vi "Moving Average Stacked Registers While Loop.vi"() -> ()   [LabVIEW 2023]
panel:
  out "Moving Average":dbl
  out "Current Value":dbl
  in  "stop":bool
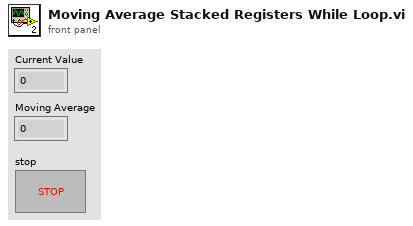
[diagram p1: front panel]
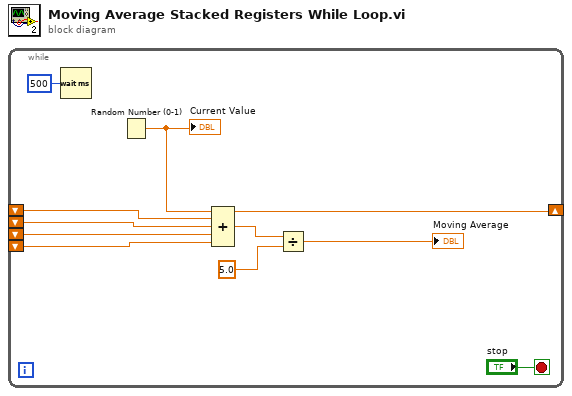
[diagram p0: block diagram]
diagram:
  n1 = while {
    shift-right: [w4] -> _
    shift-left: _ -> [w8]
    shift-left: _ -> [w6]
    shift-left: _ -> [w7]
    shift-left: _ -> [w5]
    stop <- "stop" stop-if-true
    n2 = Wait (ms)(milliseconds to wait=u32 500) -> ()  [unwired: 1 out]
    n3 = Random Number (0-1)() -> (number: 0 to 1=w4:dbl)
    "Current Value" <- w4
    n4 = Compound Arithmetic op=ADD(w4, w8, w5, w7, w6) -> (w2:dbl)
    n5 = Divide(x=w2, y=5.0) -> (x/y=→"Moving Average":dbl)
  }
